vi "校准时间.vi"() -> ()   [LabVIEW 2019]
panel:
  out "时间差":dbl
  in  "校准时间":bool
  out "计算机时间":string
  out "错误输出":errorcluster
  in  "错误输入":errorcluster
  out "VISA资源名称输出":refnum<visa-resource-name>
  out "源表时间":string
  in  "VISA资源名称":refnum<visa-resource-name>
  out "日期/时间字符串":string
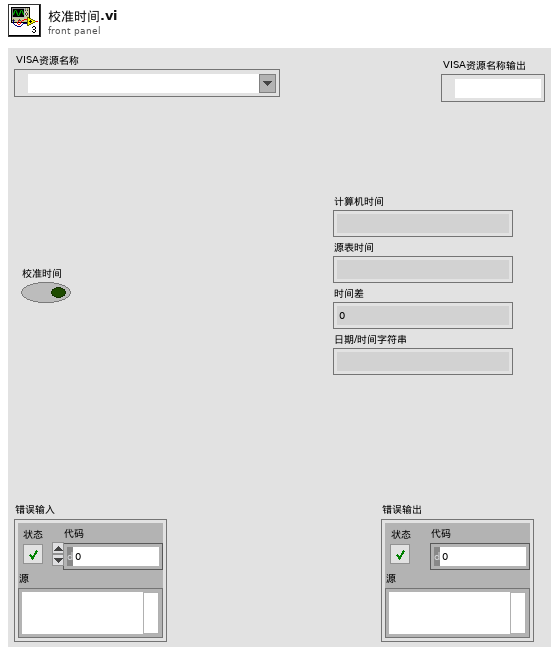
[diagram p1: front panel]
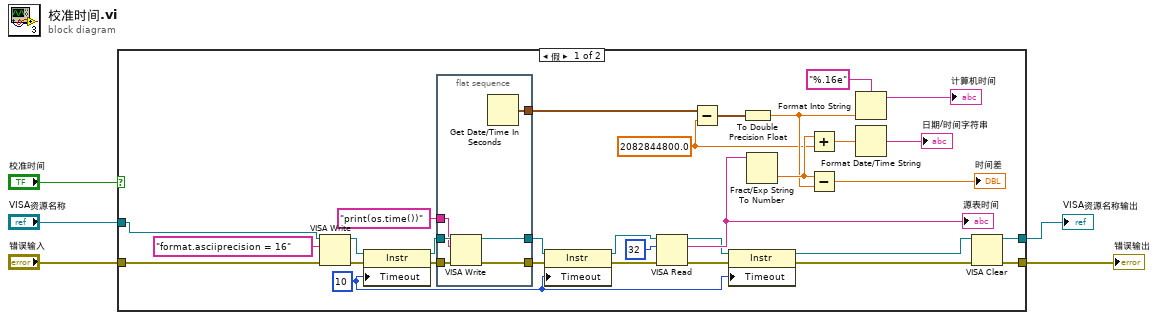
[diagram p0: block diagram]
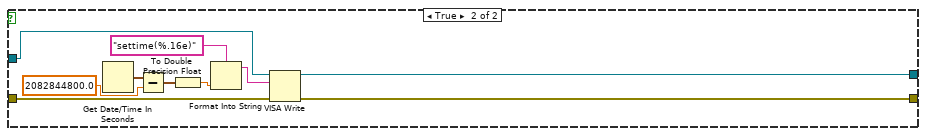
[diagram p2: hidden frame]
diagram:
  n1 = case shown="假" "校准时间" {
    tunnel: "错误输入" -> [w8 w52]
    tunnel: "VISA资源名称" -> [w9 w51]
    tunnel: [w6 w50] -> w3
    tunnel: [w7 w49] -> w4
    frame False {
      w12 = u32 10 ("General Settings:Timeout Value")
      w13 = 2082844800.0 ("x-y")
      n2 = VISA Write(VISA resource name=w9, write buffer="format.asciiprecision = 16" ("格式字符串"), error in (no error)=w8) -> (VISA resource name out=w17:refnum<visa-resource-name>, error out=w18:errorcluster)  [unwired: 1 out]
      n3 = property class="Instr"(reference=w17, error in=w18, "Timeout"=w12) -> (reference out=w27:refnum<visa-resource-name>, error out=w28:errorcluster)
      n4 = flat-sequence {
        tunnel: [w42] -> w19
        tunnel: [w41] -> w20
        tunnel: w27 -> [w40]
        tunnel: w28 -> [w39]
        tunnel: "print(os.time())" ("写入缓冲区") -> [w38]
        tunnel: [w37] -> w30
        frame #0 {
          n5 = VISA Write(VISA resource name=w40, write buffer=w38, error in (no error)=w39) -> (VISA resource name out=w42:refnum<visa-resource-name>, error out=w41:errorcluster)  [unwired: 1 out]
          n6 = Get Date/Time In Seconds() -> (seconds since 1Jan1904=w37:timestamp)
        }
      }
      n7 = property class="Instr"(reference=w19, error in=w20, "Timeout"=w12) -> (reference out=w22:refnum<visa-resource-name>, error out=w21:errorcluster)
      n8 = VISA Read(VISA resource name=w22, byte count=u32 32 ("字节总数"), error in (no error)=w21) -> (VISA resource name out=w23:refnum<visa-resource-name>, read buffer=w29:string, error out=w24:errorcluster)  [unwired: 1 out]
      "源表时间" <- w29
      n9 = Subtract(x=w30, y=w13) -> (x-y=w31:timestamp)
      n10 = property class="Instr"(reference=w23, error in=w24, "Timeout"=w12) -> (reference out=w25:refnum<visa-resource-name>, error out=w26:errorcluster)
      n11 = To Double Precision Float(number=w31) -> (double precision float=w33:dbl)
      n12 = Fract/Exp String To Number(string=w29) -> (number=w34:dbl)  [unwired: 3 in, 1 out]
      n13 = Add(x=w34, y=w13) -> (x+y=w32:dbl)
      n14 = Subtract(x=w34, y=w33) -> (x-y=→"时间差":dbl)
      n15 = Format Into String(format string="%.16e" ("格式字符串"), w33) -> (resulting string=→"计算机时间":string)  [unwired: 2 in, 1 out]
      n16 = Format Date/Time String(seconds (now)=w32) -> (date/time string=→"日期/时间字符串":string)  [unwired: 2 in]
      n17 = VISA Clear(VISA resource name=w25, error in (no error)=w26) -> (VISA resource name out=w7:refnum<visa-resource-name>, error out=w6:errorcluster)
    }
    frame True {
      n18 = Get Date/Time In Seconds() -> (seconds since 1Jan1904=w46:timestamp)
      n19 = Subtract(x=w46, y=2082844800.0 ("x-y")) -> (x-y=w47:timestamp)
      n20 = To Double Precision Float(number=w47) -> (double precision float=w48:dbl)
      n21 = Format Into String(format string="settime(%.16e)" ("格式字符串"), w48) -> (resulting string=w43:string)  [unwired: 2 in, 1 out]
      n22 = VISA Write(VISA resource name=w51, write buffer=w43, error in (no error)=w52) -> (VISA resource name out=w49:refnum<visa-resource-name>, error out=w50:errorcluster)  [unwired: 1 out]
    }
  }
  "VISA资源名称输出" <- w4
  "错误输出" <- w3
